vi "1D U64.vi"(5 "format string (%_20d)":string="%_20d", 7 "key description":string, 8 "sections":string[](array[string]), 9 "numeric":u64[](array[numeric]), 11 "info data":string) -> (0 "sections out":string[](array[string]), 3 "info data out":string)   [LabVIEW 2019, in "infolib.lvlib"]
doc: "Add a new numeric table to Info Data string. If section exists in Info Data string, inserts key into this section. If collumn vector is set to false, the result will be one long line."
uses:
  infolib.lvlib
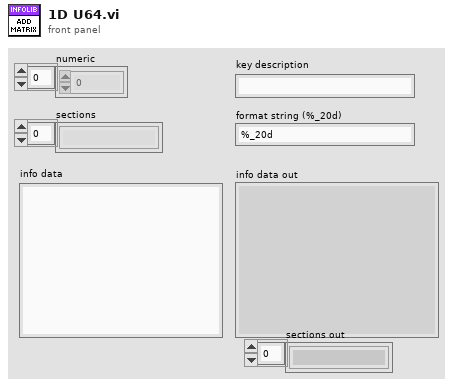
[diagram p1: front panel]
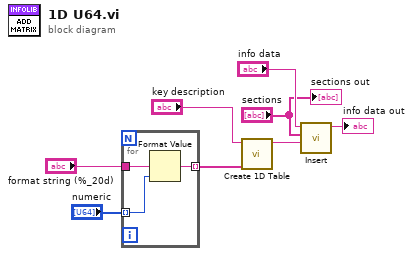
[diagram p0: block diagram]
diagram:
  n1 = for {
    tunnel: "numeric" -> [w11] mode=indexing
    tunnel: "format string (%_20d)" -> [w10]
    tunnel: [w9] -> w2 mode=indexing
    n2 = Format Value(format string=w10, value (0)=w11) -> (output string=w9:string)  [unwired: 1 in]
  }
  n3 = call "Create 1D Table.vi"("formatted values"=w2, "table name"="key description") -> ("table"=w1:string)  [unwired: 8 in, 1 out]
  n4 = call "Insert.vi"("insert"=w1, "sections"="sections", "info data"="info data") -> ("info data out"=→"info data out":string)  [unwired: 8 in]
  "sections out" <- "sections"
